vi "Actor Core.vi"(8 "error in":errorcluster, 11 "Nested in":refnum<class "Stage Controller.lvclass">) -> (0 "error out":errorcluster, 3 "Actor out":refnum<class "Actor.lvclass">)   [LabVIEW 2020, in "Stage.lvlib" / "Stage Controller.lvlib" / "Stage Controller.lvclass"]
doc: "(<B>Filename</B>: Actor Framework.lvlib:Actor.lvclass:Actor Core.vi)\n\nReceives messages to the actor, reacts to them, and initiates any error handling that may shut the actor down.\n\nDescendant classes may override this VI to append parallel tasks for the actor to complete while it handles messages. Overrides use the Call Parent Method node."
uses:
  Stage Controller.lvclass
  C:/Program Files/National Instruments/LabVIEW 2020/vi.lib/ActorFramework/Actor/Actor.lvclass
  <vilib>/ActorFramework/Actor/Actor.lvclass
  Stage Controller.lvclass/Stage Controller.ctl
  <vilib>/ActorFramework/Actor/Actor.lvclass/Actor.ctl
  <vilib>/ActorFramework/Message Enqueuer/Message Enqueuer.lvclass/Message Enqueuer.ctl
  <vilib>/ActorFramework/Message Enqueuer/Init from Existing Queue.vi
  <vilib>/ActorFramework/Message Enqueuer/Enqueue.vi
  <vilib>/ActorFramework/Stop Msg/Stop Msg.lvclass
  C:/Program Files/National Instruments/LabVIEW 2020/vi.lib/ActorFramework/Message/Message.lvclass
  <vilib>/ActorFramework/Message Priority Queue/Priority Enqueue.vi
  <vilib>/ActorFramework/Message Enqueuer/Message Enqueuer.lvclass
panel:
  in  "StageX-":bool
  in  "StageX+":bool
  in  "StageY+":bool
  in  "StageY-":bool
  in  "StageY++":bool
  in  "StageX--":bool
  in  "StageX++":bool
  in  "StageY--":bool
  in  "XYIncreatement+":dbl min=0.0 max=50.0
  in  "XYIncreatement++":dbl min=0.0 max=100.0
  in  "StageZ++":bool
  in  "StageZ--":bool
  in  "StageZ+":bool
  in  "StageZ-":bool
  # "Inc."
  # "Y"
  # "um"
  # "X"
  # "um"
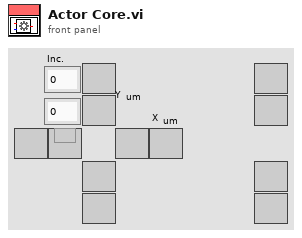
[diagram p1: front panel]
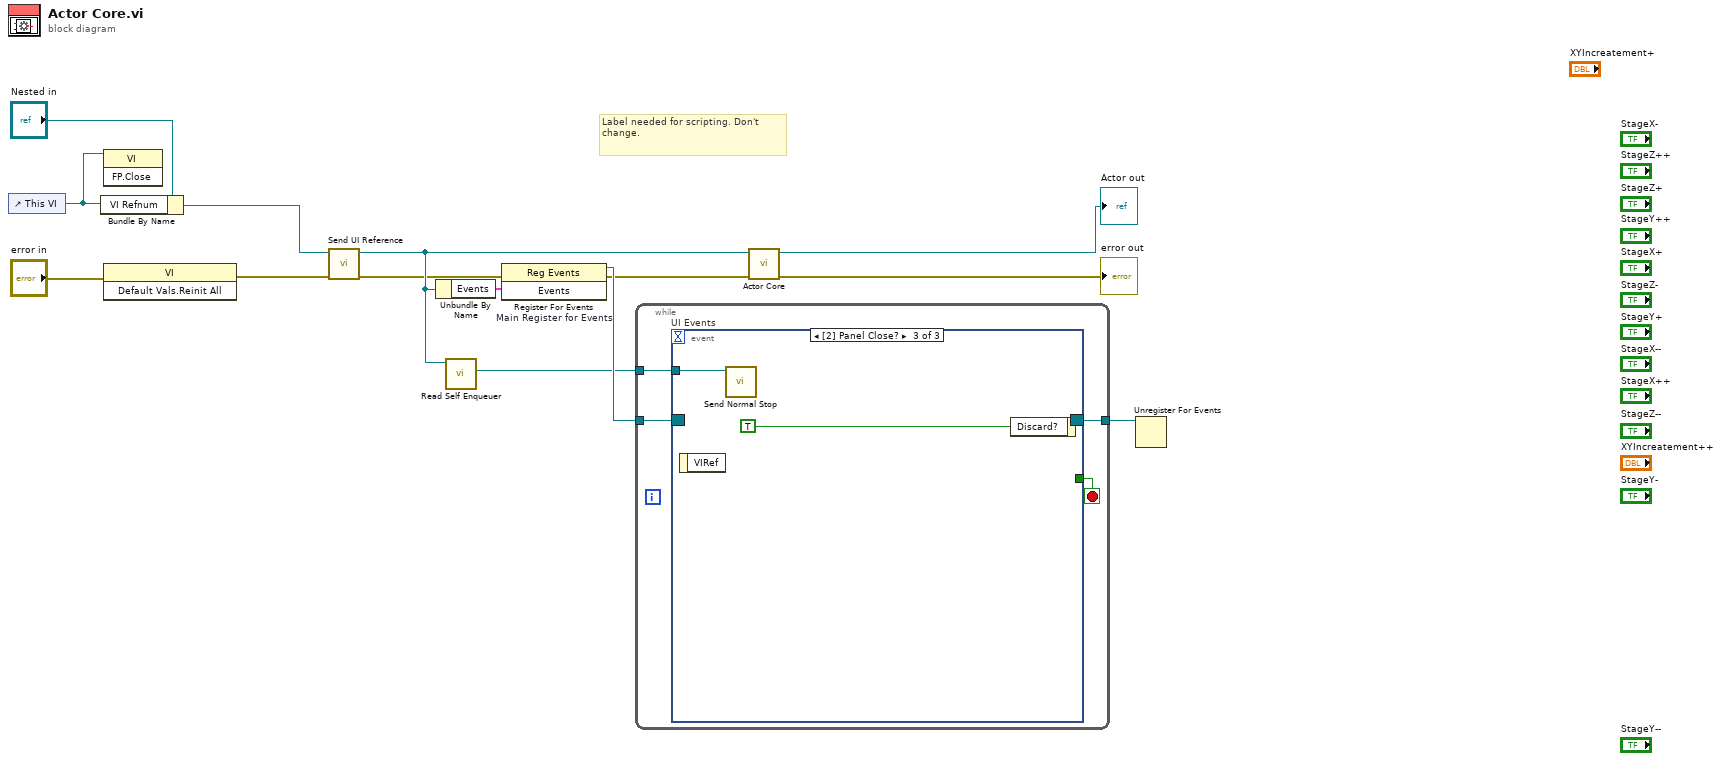
[diagram p0: block diagram]
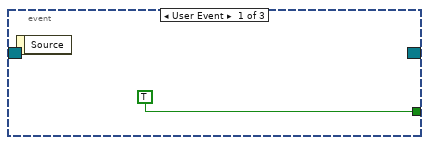
[diagram p2: hidden frame]
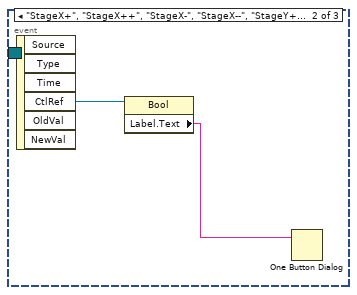
[diagram p3: hidden frame]
diagram:
  # "Label needed for scripting. Don't change."
  n1 = control-ref of="This VI"() -> (w1:refnum<vi>)
  n2 = Bundle By Name(cluster="Nested in", "VI Refnum"=w1) -> (w5:refnum<class "Stage Controller.lvclass">)
  n3 = invoke class="VI" method="FP.Close"(reference=w1) -> ()  [unwired: 2 in, 3 out]
  n4 = invoke class="VI" method="Default Vals.Reinit All"(error in="error in") -> (error out=w3:errorcluster)  [unwired: 2 in, 2 out]
  n5 = call-dynamic "Send UI Reference.vi"("error in (no error)"=w3, "Stage Controller in"=w5) -> ("error out"=w2:errorcluster, "Stage Controller out"=w4:refnum<class "Stage Controller.lvclass">)  [unwired: 8 in]
  n6 = Unbundle By Name(w4) -> ("Events"=w11:cluster{"Stop":refnum<user-event>})
  n7 = call <vilib>:"Read Self Enqueuer.vi"("Actor"=w4) -> ("Self Enqueuer"=w9:refnum<class "Message Enqueuer.lvclass">)  [unwired: 10 in]
  n8 = register-events "Main Register for Events"(error in=w2, w11) -> (reference out=w12:refnum<event-registration>, error out=w8:errorcluster)  [unwired: 1 in]
  n9 = while {
    tunnel: w12 -> [w18]
    tunnel: [w16] -> w10
    tunnel: w9 -> [w15]
    stop <- w17 stop-if-true
    n10 = event "UI Events" shown="[2] Panel Close?" {
      selector: w18 -> [_ _ _]
      dyn-events: [_ _ _] -> w16
      timeout: _ -> [_ _ _]
      tunnel: [TRUE _ _] -> w17
      tunnel: w15 -> [_ _ w22]
      event User Event {
        n11 = event-data() -> ()  [unwired: 1 in, 1 out]
      }
      event "StageX+", "StageX++", "StageX-", "StageX--", "StageY+", "StageY++", "StageY-", "StageY--", "StageZ+", "StageZ++", "StageZ-", "StageZ--": Value Change {
        n12 = event-data() -> ("CtlRef"=w21:refnum<vi>)  [unwired: 1 in, 5 out]
        n13 = property class="Bool"(reference=w21) -> ("Label.Text"=w20:string)  [unwired: 1 in, 2 out]
        n14 = One Button Dialog(message=w20) -> ()  [unwired: 1 in, 1 out]
      }
      event Panel Close? {
        n15 = event-data() -> ()  [unwired: 1 in, 1 out]
        n16 = call <vilib>:"Send Normal Stop.vi"("Message Enqueuer"=w22) -> ()  [unwired: 10 in, 1 out]
        n17 = event-data("Discard?"=TRUE) -> ()  [unwired: 1 in, 1 out]
      }
    }
  }
  n18 = call-parent "Actor Core.vi"("error in"=w8, "Actor in"=w4) -> ("error out"=→"error out":errorcluster, "Actor out"=→"Actor out":refnum<class "Actor.lvclass">)  [unwired: 8 in]
  n19 = Unregister For Events(event registration refnum=w10) -> ()  [unwired: 1 in, 1 out]
